vi "HapticSPM_write.vi"() -> ()   [LabVIEW 2021]
uses:
  <userlib>/Haptic Prog Interface/Haptic Prog Interface.lvlib
  <userlib>/Nanonis Prog Interface V5/Nanonis Prog Interface.lvlib
panel:
  in  "XY Write":bool
  out "Surface":dbl caption="Numeric" format="%#_5p"
  out "Z-Position":dbl caption="Numeric" format="%#_5p"
  out "y":string
  out "x":string
  out "scan data":dbl[][](array[numeric])
  out "2D Picture":picture
  out "Force":dbl(slide) scale=0.0..3.0
  out "Frame String":string
  in  "Stop":bool
  out "Safe tip":bool
  out "Value":dbl caption="Numeric" format="%#_2p"
  out "Reframed Position (m)":cluster{"x (m)":dbl, "y (m)":dbl, "z (m)":dbl} {"z (m)" format="%.1p"; "y (m)" format="%.1p"; "x (m)" format="%.1p"}
  out "Frame Properties (m)":T1
  in  "Function":string(combo)="0" caption="Combo Box"
  in  "Gain (mm/pm)":dbl=1.0 caption="Numeric" format="%.1g"
  in  "k":dbl=1.0 caption="Numeric" format="%.1g"
  in  "Setpoint":dbl=2.0 caption="Numeric" format="%.0p"
  in  "Gain":dbl=1.0 caption="Numeric" format="%.1g"
  out "Click Number":dbl caption="Numeric" format="%#_1g"
  in  "Write Z":bool
  in  "Planing Toggle":bool
  in  "Planing Reset":bool
  in  "Save":bool
  # "Super Ultra Mega Haptic SPM Controller 3000"
  # "Scan Window"
  # "Height"
  # "Signal"
  # "Force"
  # "Planing"
  # "Force"
  # "Surface Scale"
  # "Z Write"
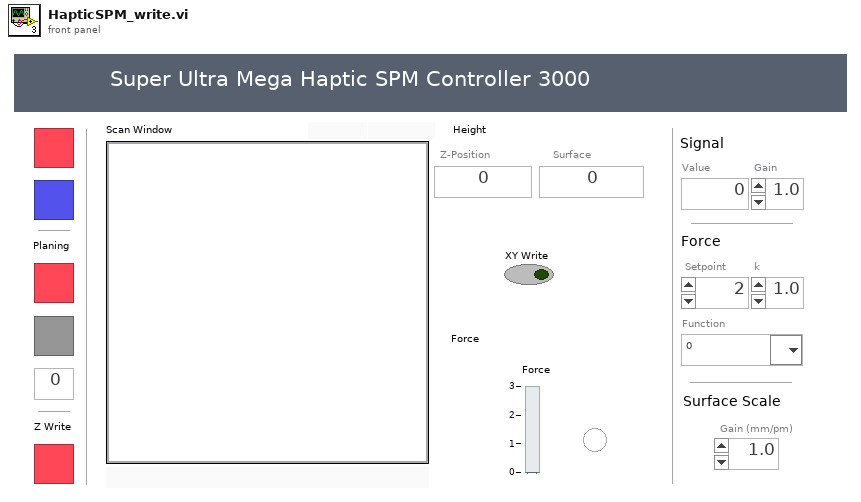
[diagram p1: front panel]
types:
  T1 = cluster{"Center coordinates (m)":cluster{"Xc":sgl, "Yc":sgl}, "Size (m)":cluster{"Width":sgl, "Height":sgl}}
  T2 = cluster{"Fx (N)":dbl, "Fy (N)":dbl, "Fz (N)":dbl}
  T3 = cluster{"kx (N/m)":dbl, "ky (N/m)":dbl, "kz (N/m)":dbl}
  T4 = cluster{"X Drag":bool, "Y Drag":bool, "Z Drag":bool}
  T5 = cluster{"x (mm)":dbl, "y (mm)":dbl, "z (mm)":dbl}
  T6 = typedef "LVBoundsTypeDef.ctl" = cluster{"Width":u32, "Height":u32}
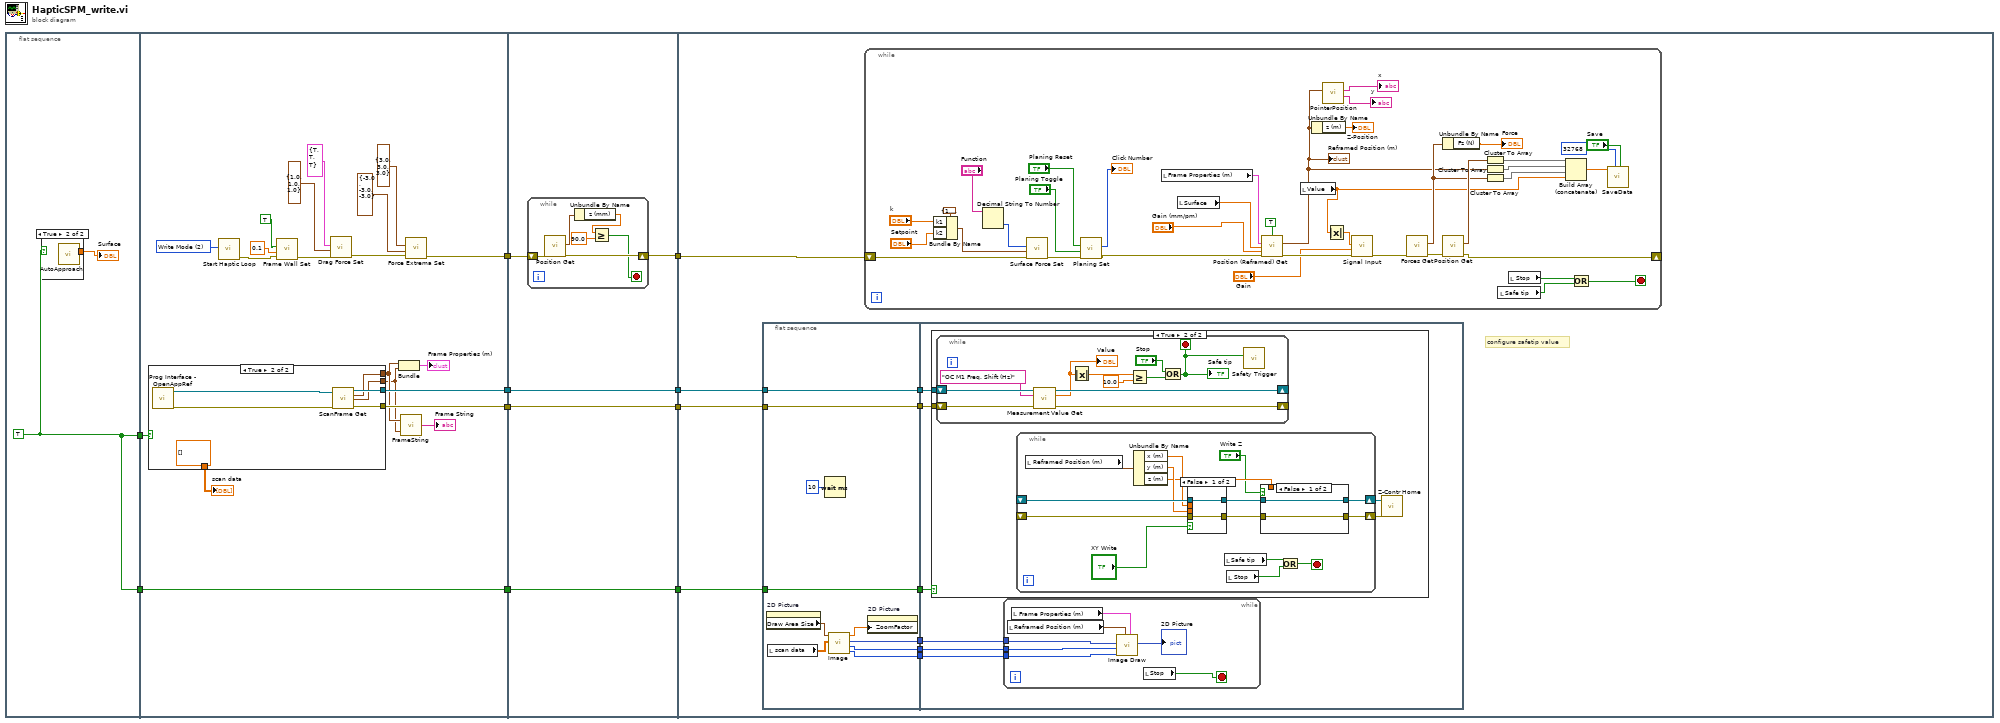
[diagram p0: block diagram]
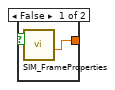
[diagram p2: hidden frame]
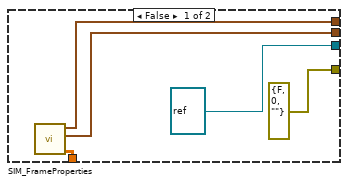
[diagram p3: hidden frame]
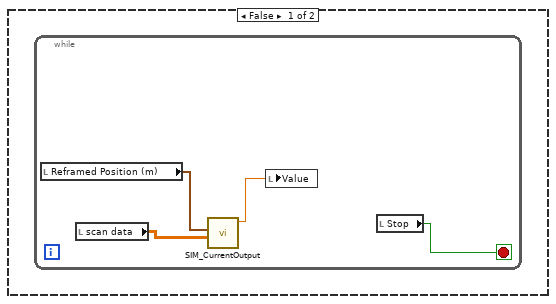
[diagram p4: hidden frame]
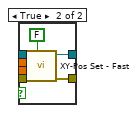
[diagram p5: hidden frame]
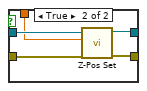
[diagram p6: hidden frame]
diagram:
  n1 = flat-sequence {
    tunnel: [w12] -> w4
    tunnel: [w12] -> w3
    tunnel: [w32] -> w10
    tunnel: [w22] -> w7
    tunnel: [w21] -> w5
    tunnel: w4 -> [w17]
    tunnel: w3 -> [w16]
    tunnel: [w16] -> w2
    tunnel: w10 -> [w51]
    tunnel: [w50] -> w9
    tunnel: [w49] -> w8
    tunnel: w7 -> [w49]
    tunnel: [w48] -> w6
    tunnel: w5 -> [w48]
    tunnel: w2 -> [w47]
    tunnel: [w47] -> w1
    tunnel: w9 -> [w67]
    tunnel: w8 -> [w65]
    tunnel: w6 -> [w63]
    tunnel: w1 -> [w62]
    frame #0 {
      w12 = TRUE
      n2 = case shown="True" w12 {
        tunnel: [w13 w14] -> w11
        frame False {
          n3 = call "SIM_FrameProperties.vi"() -> ("Surf Loc (m)"=w13:dbl)  [unwired: 8 in, 3 out]
        }
        frame True {
          n4 = call "AutoApproach.vi"() -> ("Surface Location (m)"=w14:dbl)  [unwired: 11 in]
        }
      }
      "Surface" <- w11
    }
    frame #1 {
      w34 = u16 2 items=["Custom Mode", "Read Mode", "Write Mode"] ("Mode Selection")
      n5 = case shown="True" w17 {
        tunnel: [refnum<vi> refnum ("Application ref out") w46] -> w22
        tunnel: [errorcluster {"status"=FALSE, "code"=0, "source"=""} ("error out") w45] -> w21
        tunnel: [w37 w44] -> w20
        tunnel: [w36 w43] -> w19
        tunnel: [w35 dbl[][] [] ("data")] -> w15
        frame False {
          n6 = call "SIM_FrameProperties.vi"() -> ("data"=w35:dbl[][], "Size (m)"=w36:cluster{"Width":sgl, "Height":sgl}, "Center coordinates (m)"=w37:cluster{"Xc":sgl, "Yc":sgl})  [unwired: 8 in, 1 out]
        }
        frame True {
          n7 = call <userlib>:"Prog Interface - OpenAppRef.vi"() -> ("Error out"=w40:errorcluster, "Application reference"=w41:refnum<vi>)  [unwired: 6 in]
          n8 = call <userlib>:"ScanFrame Get.vi"("Application ref in"=w41, "error in (no error)"=w40) -> ("Application ref out"=w46:refnum<vi>, "Center coordinates (m)"=w44:cluster{"Xc":sgl, "Yc":sgl}, "Size (m)"=w43:cluster{"Width":sgl, "Height":sgl}, "error out"=w45:errorcluster)  [unwired: 9 in, 1 out]
        }
      }
      "scan data" <- w15
      n9 = call <userlib>:"Start Haptic Loop.vi"("Mode Selection"=w34) -> ("error out"=w25:errorcluster)  [unwired: 10 in]
      n10 = call <userlib>:"Frame Wall Set.vi"("error in (no error)"=w25, "Wall Stiffness (N/m)"=0.1 ("Wall Stiffness"), "Restrict to Frame"=TRUE) -> ("error out"=w24:errorcluster)  [unwired: 8 in]
      n11 = call <userlib>:"Drag Force Set.vi"("error in (no error)"=w24, "Drag Coefficients (N/m)"=T3 {"kx (N/m)"=1.0, "ky (N/m)"=1.0, "kz (N/m)"=1.0} ("Drag Coefficients"), "Drag Force Toggles"=T4 {"X Drag"=TRUE, "Y Drag"=TRUE, "Z Drag"=TRUE}) -> ("error out"=w33:errorcluster)  [unwired: 8 in]
      n12 = Bundle("Center coordinates (m)"=w20, "Size (m)"=w19) -> (→"Frame Properties (m)":T1)  [unwired: 1 in]
      n13 = call "FrameString.vi"("Size (m)"=w19, "Center coordinates (m)"=w20) -> ("string"=→"Frame String":string)
      n14 = call <userlib>:"Force Extrema Set.vi"("error in (no error)"=w33, "Minimum Force (N)"=T2 {"Fx (N)"=-3.0, "Fy (N)"=-3.0, "Fz (N)"=-3.0} ("Minimum Force"), "Maximum Force (N)"=T2 {"Fx (N)"=3.0, "Fy (N)"=3.0, "Fz (N)"=3.0} ("Maximum Force")) -> ("error out"=w32:errorcluster)  [unwired: 8 in]
    }
    frame #2 {
      n15 = while {
        shift-right: [w56] -> w50
        shift-left: w51 -> [w57]
        stop <- w52 stop-if-true
        n16 = call <userlib>:"Position Get.vi"("error in (no error)"=w57) -> ("error out"=w56:errorcluster, "Position"=w55:T5)  [unwired: 9 in]
        n17 = Unbundle By Name(w55) -> ("z (mm)"=w54:dbl)
        n18 = Greater Or Equal?(x=w54, y=90.0) -> (x >= y?=w52:bool)
      }
    }
    frame #3 {
      # "configure safetip value"
      n19 = flat-sequence {
        tunnel: [w76] -> w66
        tunnel: w65 -> [w76]
        tunnel: [w75] -> w64
        tunnel: w63 -> [w75]
        tunnel: w62 -> [w74]
        tunnel: [w74] -> w61
        tunnel: [w70] -> w60
        tunnel: [w69] -> w59
        tunnel: [w68] -> w58
        tunnel: w66 -> [w83]
        tunnel: w64 -> [w82]
        tunnel: w61 -> [w81]
        tunnel: w60 -> [w80]
        tunnel: w59 -> [w79]
        tunnel: w58 -> [w78]
        frame #0 {
          n20 = property on="2D Picture" class="Pict"() -> ("Draw Area Size"=w73:T6)  [unwired: 2 in, 2 out]
          n21 = local read "scan data"() -> (w71:dbl[][])
          n22 = Wait (ms)(milliseconds to wait=u32 10) -> ()  [unwired: 1 out]
          n23 = call "Image.vi"("data"=w71, "Draw Area Size"=w73) -> ("Rectangle.bottom"=w68:i16, "Rectangle.right"=w69:i16, "new picture"=w70:picture, "ZoomFactor"=w72:dbl)  [unwired: 6 in]
          n24 = property on="2D Picture" class="Pict"("ZoomFactor"=w72) -> ()  [unwired: 2 in, 2 out]
        }
        frame #1 {
          n25 = case shown="True" w81 {
            tunnel: w83 -> [_ w98]
            tunnel: w82 -> [_ w97]
            frame False {
              n26 = while {
                stop <- w92 stop-if-true
                n27 = local read "Reframed Position (m)"() -> (w93:cluster{"x (m)":dbl, "y (m)":dbl, "z (m)":dbl})
                n28 = local read "scan data"() -> (w91:dbl[][])
                n29 = call "SIM_CurrentOutput.vi"("array"=w91, 10:w93) -> ("Current Out (A)"=w94:dbl)  [unwired: 8 in, 1 out]
                n30 = local write "Value"(w94) -> ()
                n31 = local read "Stop"() -> (w92:bool)
              }
            }
            frame True {
              n32 = while {
                shift-right: [w107] -> _
                shift-left: w98 -> [w109]
                shift-right: [w106] -> _
                shift-left: w97 -> [w108]
                stop <- w102 stop-if-true
                n33 = call <userlib>:"Measurement Value Get.vi"("error in (no error)"=w108, "Signal Name"="OC M1 Freq. Shift (Hz)", "Application ref in"=w109) -> ("error out"=w106:errorcluster, "Measurement value"=w99:sgl, "Application ref out"=w107:refnum<vi>)  [unwired: 5 in]
                "Value" <- w99
                n34 = Absolute Value(x=w99) -> (abs(x)=w101:sgl)
                n35 = Greater Or Equal?(x=w101, y=sgl 10.0) -> (x >= y?=w104:bool)
                n36 = Or(x="Stop", y=w104) -> (x .or. y?=w102:bool)
                "Safe tip" <- w102
                n37 = call <userlib>:"Safety Trigger.vi"("Safety Trigger"=w102) -> ()  [unwired: 9 in, 2 out]
              }
              n38 = while {
                shift-right: [w119] -> w96
                shift-left: _ -> [w123]
                shift-right: [w117] -> w95
                shift-left: _ -> [w124]
                stop <- w112 stop-if-true
                n39 = local read "Reframed Position (m)"() -> (w122:cluster{"x (m)":dbl, "y (m)":dbl, "z (m)":dbl})
                n40 = Unbundle By Name(w122) -> ("x (m)"=w121:dbl, "y (m)"=w120:dbl, "z (m)"=w115:dbl)
                n41 = case shown="False" "XY Write" {
                  tunnel: w124 -> [w125 w133]
                  tunnel: w123 -> [w126 w132]
                  tunnel: w121 -> [_ w131]
                  tunnel: w120 -> [_ w130]
                  tunnel: [w126 w128] -> w118
                  tunnel: [w125 w127] -> w116
                  frame False {
                  }
                  frame True {
                    n42 = call <userlib>:"XY-Pos Set - Fast.vi"("Wait end-of-motion (T=True)"=FALSE, "error in (no error)"=w133, "Y (m)"=w130, "X (m)"=w131, "Application ref in"=w132) -> ("error out"=w127:errorcluster, "Application ref out"=w128:refnum<vi>)  [unwired: 4 in]
                  }
                }
                n43 = local read "Safe tip"() -> (w114:bool)
                n44 = local read "Stop"() -> (w113:bool)
                n45 = case shown="False" "Write Z" {
                  tunnel: [w135 w138] -> w119
                  tunnel: w118 -> [w135 w140]
                  tunnel: [w134 w137] -> w117
                  tunnel: w116 -> [w134 w139]
                  tunnel: w115 -> [_ w136]
                  frame False {
                  }
                  frame True {
                    n46 = call <userlib>:"Z-Pos Set.vi"("error in (no error)"=w139, "Z position (m)"=w136, "Application ref in"=w140) -> ("error out"=w137:errorcluster, "Application ref out"=w138:refnum<vi>)  [unwired: 7 in]
                  }
                }
                n47 = Or(x=w114, y=w113) -> (x .or. y?=w112:bool)
              }
              n48 = call <userlib>:"Z-Contr Home.vi"("Error in (no error)"=w95, "Application ref in"=w96) -> ()  [unwired: 8 in, 2 out]
            }
          }
          n49 = while {
            tunnel: w80 -> [w89]
            tunnel: w79 -> [w88]
            tunnel: w78 -> [w87]
            stop <- w90 stop-if-true
            n50 = local read "Reframed Position (m)"() -> (w86:cluster{"x (m)":dbl, "y (m)":dbl, "z (m)":dbl})
            n51 = local read "Frame Properties (m)"() -> (w85:T1)
            n52 = call "Image Draw.vi"("Frame Properties (m)"=w85, "Reframed Position (m)"=w86, "ih"=w87, "iw"=w88, "picture"=w89) -> ("new picture"=→"2D Picture":picture)  [unwired: 6 in]
            n53 = local read "Stop"() -> (w90:bool)
          }
        }
      }
      n54 = while {
        shift-right: [w172] -> _
        shift-left: w67 -> [w179]
        stop <- w151 stop-if-true
        n55 = Bundle By Name(cluster=cluster{"k1":dbl, "k2":dbl, "k3":dbl, "k4":dbl} {"k1"=1.0, "k2"=1.0, "k3"=1.0, "k4"=1.0} ("Force Constants"), "k1"="k", "k2"="Setpoint") -> (w165:cluster{"k1":dbl, "k2":dbl, "k3":dbl, "k4":dbl})
        n56 = Decimal String To Number(string="Function") -> (number=w162:i32)  [unwired: 2 in, 1 out]
        n57 = call <userlib>:"Surface Force Set.vi"("error in (no error)"=w179, "Force Constants"=w165, "Force Settings"=w162) -> ("error out"=w178:errorcluster)  [unwired: 8 in]
        n58 = call <userlib>:"Planing Set.vi"("error in (no error)"=w178, "Planing"="Planing Toggle", "Reset"="Planing Reset") -> ("error out"=w168:errorcluster, "Number of Clicks"=→"Click Number":i8)  [unwired: 7 in]
        n59 = local read "Frame Properties (m)"() -> (w149:T1)
        n60 = local read "Surface"() -> (w176:dbl)
        n61 = call <userlib>:"Position (Reframed) Get.vi"("Z Rescaling"=TRUE, "Frame Properties (m)"=w149, "Surface Location (m)"=w176, "Scaling (mm per pm)"="Gain (mm/pm)", "error in (no error)"=w168) -> ("Reframed Position (m)"=w145:cluster{"x (m)":dbl, "y (m)":dbl, "z (m)":dbl}, "error out"=w174:errorcluster)  [unwired: 9 in]
        "Reframed Position (m)" <- w145
        n62 = local read "Value"() -> (w141:dbl)
        n63 = Unbundle By Name(w145) -> ("z (m)"=→"Z-Position":dbl)
        n64 = call "PointerPosition.vi"("Reframed Position (m)"=w145) -> ("y string"=→"y":string, "x string"=→"x":string)  [unwired: 9 in]
        n65 = Absolute Value(x=w141) -> (abs(x)=w142:dbl)
        n66 = call <userlib>:"Signal Input.vi"("error in (no error)"=w174, "Gain"="Gain", "Signal"=w142) -> ("error out"=w175:errorcluster)  [unwired: 8 in]
        n67 = call <userlib>:"Forces Get.vi"("error in (no error)"=w175) -> ("error out"=w173:errorcluster, "Force (N)"=w150:T2)  [unwired: 9 in]
        n68 = call <userlib>:"Position Get.vi"("error in (no error)"=w173) -> ("error out"=w172:errorcluster, "Position"=w159:T5)  [unwired: 9 in]
        n69 = Unbundle By Name(w150) -> ("Fz (N)"=→"Force":dbl)
        n70 = Cluster To Array(cluster=w159) -> (array=w158:dbl[])
        n71 = Cluster To Array(cluster=w145) -> (array=w157:dbl[])
        n72 = Cluster To Array(cluster=w150) -> (array=w156:dbl[])
        n73 = local read "Safe tip"() -> (w152:bool)
        n74 = local read "Stop"() -> (w153:bool)
        n75 = Build Array (concatenate)(w158, w157, w156, w141) -> (w155:dbl[])
        n76 = Or(x=w153, y=w152) -> (x .or. y?=w151:bool)
        n77 = call "SaveData.vi"("Save"="Save", "# Sample Points"=32768, "Data"=w155) -> ()  [unwired: 9 in]
      }
    }
  }
